vi "PH_DeformableMirror.Set Status.vi"(0 "i ref in":refnum<vi>, 5 "error in":errorcluster) -> (14 "i ref out":refnum<vi>, 19 "error out":errorcluster)   [LabVIEW 2014, in "PH_DeformableMirror.lvlib"]
uses:
  PH_DeformableMirror.lvlib
  PH_Basics/PH_StatusHandler/PH_StatusHandler.Status.ctl
  CSlibraries-extern/shs/packages/dmdriver/DMirrorBase/DMirrorBase.lvclass/DMirrorBase.ctl
  CSlibraries-extern/shs/packages/dmdriver/DMirrorBase/Is HV on.vi
  CSlibraries-extern/shs/packages/dmdriver/DMirrorBase/IsInitialized.vi
  PH_Basics/PH_StatusHandler/PH_StatusHandler.lvlib
  PH_Basics/PH_Common/PH_Common.lvlib
  CSlibraries-extern/shs/packages/dmdriver/DMirrorBase/DMirrorBase.lvclass
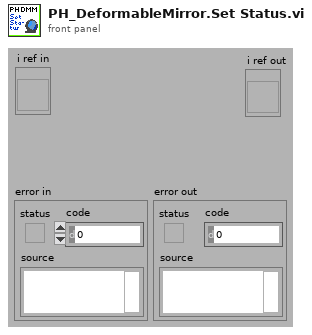
[diagram p1: front panel]
types:
  T1 = typedef "PH_StatusHandler.lvlib/PH_StatusHandler.Status.ctl" = i16
  T2 = typedef "PH_DeformableMirror.lvlib/PH_DeformableMirror.i attribute.ctl" = cluster{"DMirror.lvlib:DMirrorBase.lvclass":refnum<class "DMirrorBase.lvclass">, "Device error":errorcluster, "GUI Refs":cluster{"Delete":refnum<vi>, "Device Error":refnum<vi>, "HV on":refnum<vi>, "Channel":refnum<vi>, "Voltage":refnum<vi>, "Channel Voltages":refnum<vi>}}
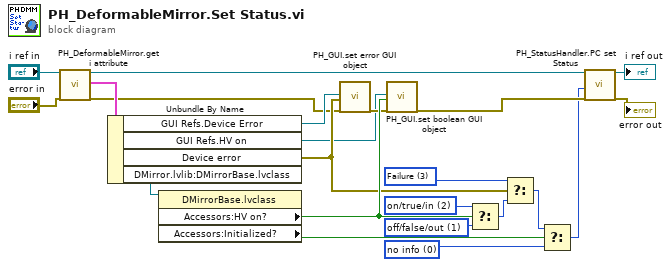
[diagram p0: block diagram]
diagram:
  w12 = T1 0 items=["no info", "off/false/out", "on/true/in", "Failure", "Alarm", "Status 1", "Status 2", "Status 3"] ("f")
  w17 = T1 1 items=["no info", "off/false/out", "on/true/in", "Failure", "Alarm", "Status 1", "Status 2", "Status 3"] ("Status")
  w16 = T1 2 items=["no info", "off/false/out", "on/true/in", "Failure", "Alarm", "Status 1", "Status 2", "Status 3"] ("Status")
  w19 = T1 3 items=["no info", "off/false/out", "on/true/in", "Failure", "Alarm", "Status 1", "Status 2", "Status 3"] ("Status")
  n1 = call "PH_DeformableMirror.get i attribute.vi"("i ref in"="i ref in", "error in (no error)"="error in") -> ("i ref out"=w2:refnum<vi>, "i attribute"=w20:T2, "error out"=w7:errorcluster)  [unwired: 15 in]
  n2 = Unbundle By Name(w20) -> ("GUI Refs.Device Error"=w8:refnum<vi>, "GUI Refs.HV on"=w5:refnum<vi>, "Device error"=w10:errorcluster, "DMirror.lvlib:DMirrorBase.lvclass"=w15:refnum<class "DMirrorBase.lvclass">)
  n3 = property class="DMirrorBase.lvclass"(reference=w15) -> ("Accessors:HV on?"=w11:bool, "Accessors:Initialized?"=w14:bool)  [unwired: 1 in, 2 out]
  n4 = call "PH_GUI.set error GUI object.vi"("GUI Refs.Device Error"=w8, "error to set"=w10, "error in (no error)"=w7) -> ("error out"=w6:errorcluster)  [unwired: 16 in]
  n5 = call "PH_GUI.set boolean GUI object.vi"("Boolean Knob GUI Ref"=w5, "Value"=w11, "error in (no error)"=w6) -> ("error out"=w4:errorcluster)  [unwired: 16 in]
  n6 = Select(t=w16, s=w11, f=w17) -> (s? t:f=w18:T1)
  n7 = Select(t=w19, s=w10, f=w18) -> (s? t:f=w13:T1)
  n8 = Select(t=w13, s=w14, f=w12) -> (s? t:f=w3:T1)
  n9 = call "PH_StatusHandler.PC set Status.vi"("i ref in"=w2, "Status"=w3, "error in (no error)"=w4) -> ("i ref out"=→"i ref out":refnum<vi>, "error out"=→"error out":errorcluster)  [unwired: 15 in]
